vi "Save.vi"(7 "Flattened String":string, 8 "error in (no error)":errorcluster, 9 "File Name":string, 10 "Folder":path, 11 "XML in":refnum<class "XML.lvclass">) -> (0 "error out":errorcluster, 3 "XML out":refnum<class "XML.lvclass">)   [LabVIEW 2020, in "XML.lvlib" / "XML.lvclass"]
uses:
  <vilib>/gpm_packages/@cs/persistence/source/XML/XML.lvclass
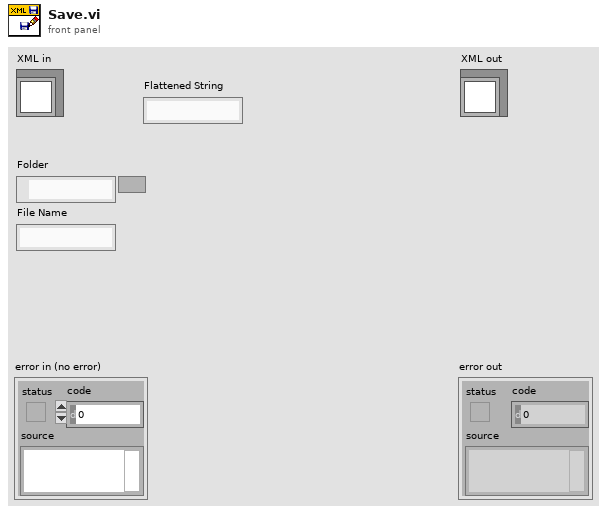
[diagram p1: front panel]
types:
  T1 = enum16{"open", "replace", "create", "open or create", "replace or create", "replace or create with confirmation"}
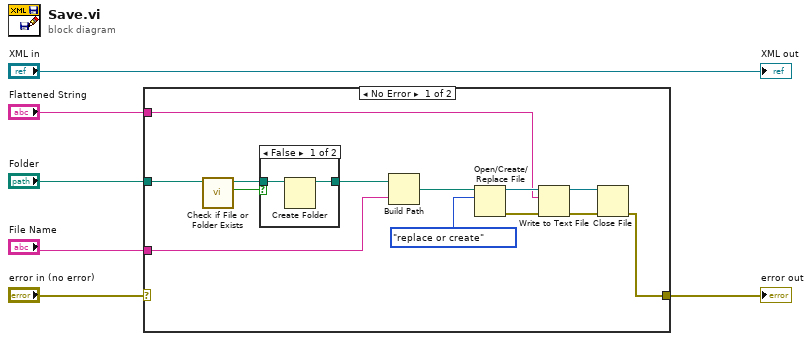
[diagram p0: block diagram]
diagram:
  n1 = case shown="No Error" "error in (no error)" {
    selector: "error in (no error)" -> [_ w23]
    tunnel: "Flattened String" -> [w10 _]
    tunnel: "Folder" -> [w9 _]
    tunnel: "File Name" -> [w8 _]
    tunnel: [w7 w23] -> w1
    frame No Error {
      n2 = call <vilib>:"Check if File or Folder Exists.vi"("path"=w9) -> ("file or folder exists?"=w12:bool, "dup path"=w13:path)  [unwired: 8 in, 1 out]
      n3 = case shown="False" w12 {
        tunnel: w13 -> [w21 w22]
        tunnel: [w20 w22] -> w14
        frame False {
          n4 = Create Folder(path (use dialog)=w21) -> (created path=w20:path)  [unwired: 2 in, 2 out]
        }
        frame True {
        }
      }
      n5 = Build Path(base path=w14, name or relative path=w8) -> (appended path=w11:path)
      n6 = Open/Create/Replace File(file path (use dialog)=w11, operation (0:open)=T1."replace or create") -> (refnum out=w16:refnum<file>, error out=w18:errorcluster)  [unwired: 4 in, 1 out]
      n7 = Write to Text File(file (use dialog)=w16, text=w10, error in=w18) -> (refnum out=w17:refnum<file>, error out=w19:errorcluster)  [unwired: 1 in, 1 out]
      n8 = Close File(refnum=w17, error in=w19) -> (error out=w7:errorcluster)  [unwired: 1 out]
    }
    frame Error {
    }
  }
  "error out" <- w1
  "XML out" <- "XML in"
